vi "MotionMagicVelocityVoltage Setter.vi"(0 "LimitReverseMotion":bool, 1 "EnableFOC":bool=TRUE, 2 "Slot":i32, 3 "Update Frequency (Hz)":dbl=100.0, 5 "StopSendingOtherRequests":bool=TRUE, 7 "Velocity":dbl, 9 "Acceleration":dbl, 12 "FeedForward":dbl, 13 "OverrideBrakeDurNeutral":bool) -> (4 "DeviceReference Out":T1)   [LabVIEW 2023]
doc: "Requests Motion Magic® to target a final velocity using a motion profile. This allows smooth transitions between velocity set points. Users can optionally provide a voltage feedforward.\nMotion Magic® Velocity produces a motion profile in real-time while attempting to honor the specified Acceleration and Jerk value. This control mode does not use the CruiseVelocity, Expo_kV, or Expo_kA configs. If the specified acceleration is zero, the Acceleration under Motion Magic® configuration parameter is used instead. This allows for runtime adjustment of acceleration for advanced users. Jerk is also specified in the Motion Magic® persistent configuration values. If Jerk is set to zero, Motion Magic® will produce a trapezoidal acceleration profile. Target velocity can also be changed on-the-fly and Motion Magic® will do its best to adjust the profile. This control mode is voltage-based, so relevant closed-loop gains will use Volts for the numerator."
uses:
  Users/Cory/Documents/PhoenixPro-LabVIEW-Generation/controls/DeviceReference.ctl
panel:
  in  "LimitForwardMotion":bool
  in  "DeviceReference":T1
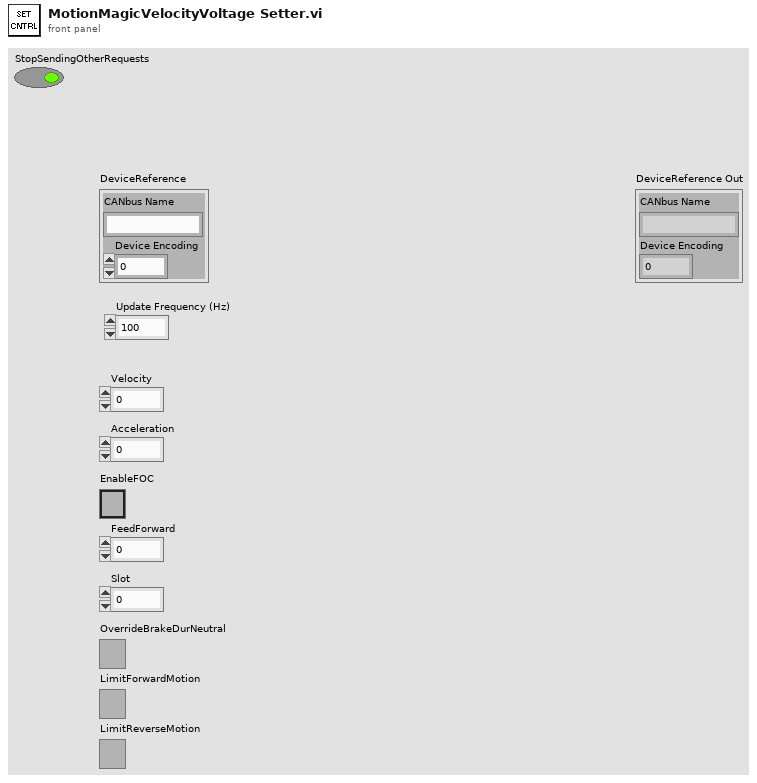
[diagram p1: front panel]
types:
  T1 = typedef "DeviceReference.ctl" = cluster{"CANbus Name":string, "Device Encoding":u32}
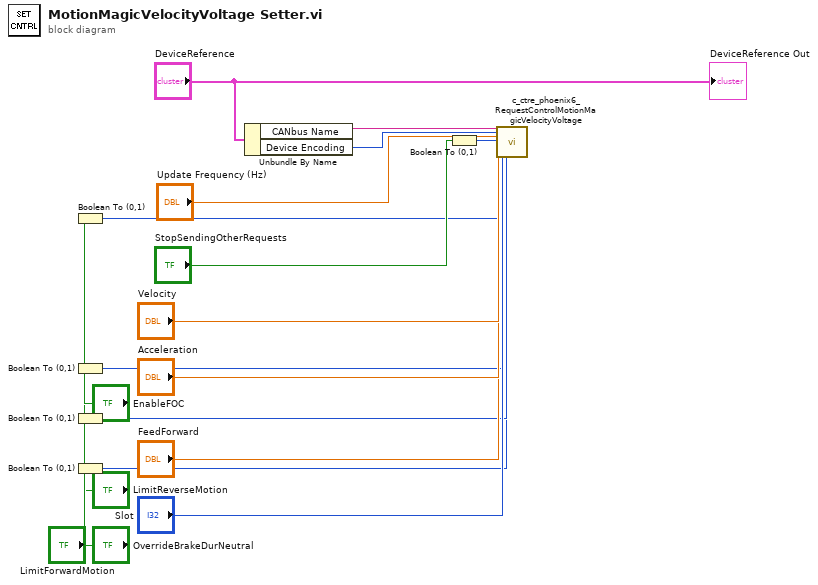
[diagram p0: block diagram]
diagram:
  n1 = Boolean To (0,1)(Boolean="EnableFOC") -> (0, 1=w9:i16)
  n2 = Boolean To (0,1)(Boolean="OverrideBrakeDurNeutral") -> (0, 1=w5:i16)
  n3 = Boolean To (0,1)(Boolean="LimitForwardMotion") -> (0, 1=w3:i16)
  n4 = Boolean To (0,1)(Boolean="LimitReverseMotion") -> (0, 1=w1:i16)
  n5 = Unbundle By Name("DeviceReference") -> ("CANbus Name"=w17:string, "Device Encoding"=w16:u32)
  n6 = Boolean To (0,1)(Boolean="StopSendingOtherRequests") -> (0, 1=w13:i16)
  n7 = call <vilib>:"c_ctre_phoenix6_RequestControlMotionMagicVelocityVoltage.vi"("String 2"=w17, "Numeric 2"=w16, "Numeric 3"="Update Frequency (Hz)", "Numeric 4"=w13, "Numeric 5"="Velocity", "Numeric 6"="Acceleration", "Numeric 7"=w9, "Numeric 8"="FeedForward", "Numeric 9"="Slot", "Numeric 10"=w5, "Numeric 11"=w3, "Numeric 12"=w1) -> ()  [unwired: 14 in, 2 out]
  "DeviceReference Out" <- "DeviceReference"
